vi "DIO sample.vi"() -> ()   [LabVIEW 2012]
doc: "Digital IO Example Program"
uses:
  Controls/DIO_bytemask.ctl
  Controls/DIO_bitMask.ctl
  OpenG SuBVIs/Variant Changed__ogtk.vi
panel:
  in  "ReInit":bool
  in  "Out Mask":T1
  in  "Tri State":enum8{"False", "True"}(ring)
  in  "stop":bool
  out "Digital Pins (Row = Byte, Column = bits, LSB on left)":bool[][](array[boolean])
  in  "Device Index":i32 max=32
  in  "OutBytes":T2 {"Out Byte 3" format="%08b"; "Out Byte 2" format="%08b"; "Out Byte 1" format="%08b"; "Out Byte 0" format="%08b"}
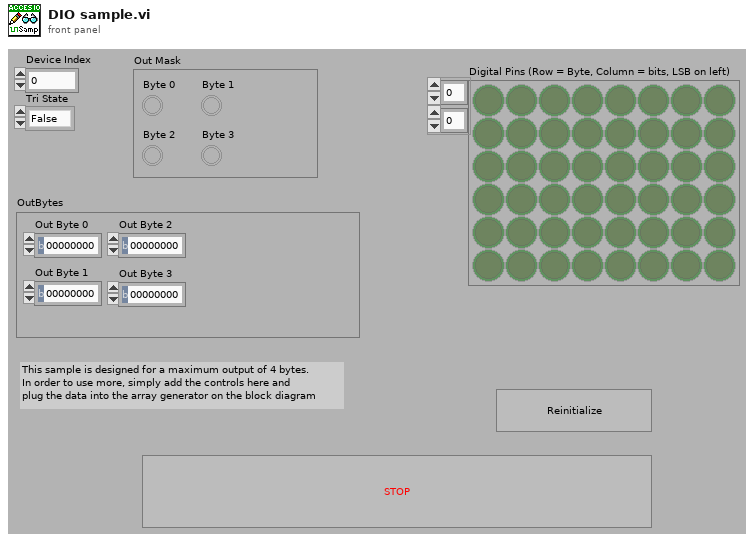
[diagram p1: front panel]
types:
  T1 = typedef "DIO_bitMask.ctl" = cluster{"Byte 0":bool, "Byte 1":bool, "Byte 2":bool, "Byte 3":bool}
  T2 = typedef "DIO_bytemask.ctl" = cluster{"Out Byte 0":u8, "Out Byte 1":u8, "Out Byte 2":u8, "Out Byte 3":u8}
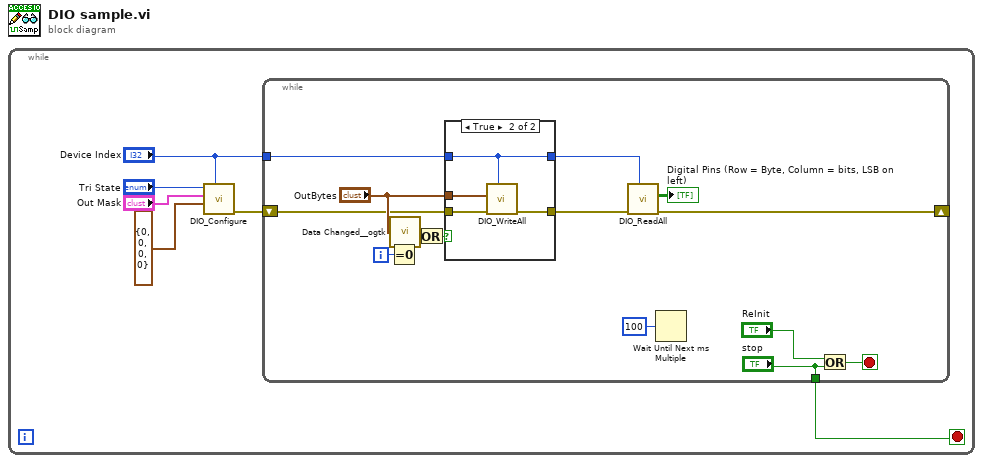
[diagram p0: block diagram]
diagram:
  n1 = while {
    stop <- w1 stop-if-true
    n2 = call "DIO_Configure.vi"("Device Index"="Device Index", "OutBytes"=T2 {"Out Byte 0"=0, "Out Byte 1"=0, "Out Byte 2"=0, "Out Byte 3"=0}, "Out Mask"="Out Mask", "Tri State"="Tri State") -> ("error out"=w6:errorcluster)  [unwired: 7 in]
    n3 = while {
      tunnel: "Device Index" -> [w17]
      shift-right: [w16] -> _
      shift-left: w6 -> [w18]
      tunnel: ["stop"] -> w1
      i -> [w8]
      stop <- w15 stop-if-true
      n4 = Equal To 0?(x=w8) -> (x = 0?=w9:bool)
      n5 = call-poly "Data Changed__ogtk.vi"("Variant"="OutBytes") -> ("Changed"=w10:bool)
      n6 = Or(x=w10, y=w9) -> (x .or. y?=w11:bool)
      n7 = case shown="True" w11 {
        tunnel: "OutBytes" -> [_ w27]
        tunnel: w18 -> [w23 w26]
        tunnel: [w23 w25] -> w20
        tunnel: w17 -> [w22 w24]
        tunnel: [w22 w24] -> w7
        frame False {
        }
        frame True {
          n8 = call "DIO_WriteAll.vi"("DeviceIndex"=w24, "error in (no error)"=w26, "OutBytes"=w27) -> ("error out"=w25:errorcluster)  [unwired: 8 in]
        }
      }
      n9 = call "DIO_ReadAll.vi"("Device Index"=w7, "error in (no error)"=w20) -> ("error out"=w16:errorcluster, "Boolean array"=→"Digital Pins (Row = Byte, Column = bits, LSB on left)":bool[][])  [unwired: 7 in, 1 out]
      n10 = Wait Until Next ms Multiple(millisecond multiple=u32 100) -> ()  [unwired: 1 out]
      n11 = Or(x="ReInit", y="stop") -> (x .or. y?=w15:bool)
    }
  }
